vi "PV Calc.vi"(8 "error in (no error)":errorcluster, 11 "LimitControl in":refnum<class "LimitControl.lvclass">) -> (0 "error out":errorcluster, 3 "LimitControl out":refnum<class "LimitControl.lvclass">)   [LabVIEW 2020, in "VolatusControl.lvlib" / "LimitControl.lvclass"]
uses:
  LimitControl.lvclass
  LimitControl.lvclass/LimitControl.ctl
  lv-vecto/Vecto/Channel DBL/Channel DBL.lvclass/Channel DBL.ctl
  <vilib>/Analysis/baseanly.llb/Mean (DBL).vi
  lv-vecto/Vecto/Group DBL/Value by Index.vi
  lv-vecto/Vecto/Channel DBL/Channel DBL.lvclass
  <vilib>/Analysis/NI_AALBase.lvlib
panel:
  out "PV":dbl
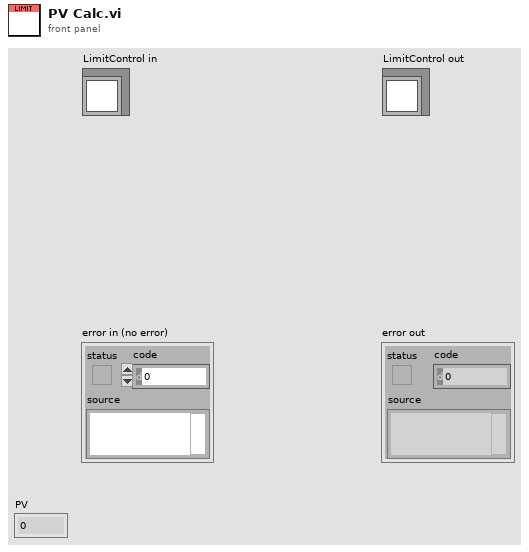
[diagram p1: front panel]
types:
  T1 = typedef "VolatusControl.lvlib/LimitControl.lvclass/PV Calc.ctl" = enum16{"Average", "Median"}
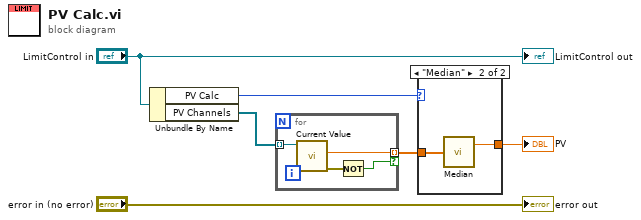
[diagram p0: block diagram]
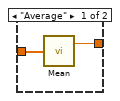
[diagram p2: hidden frame]
diagram:
  n1 = Unbundle By Name("LimitControl in") -> ("PV Calc"=w3:T1, "PV Channels"=w5:refnum<class "Channel DBL.lvclass">[])
  n2 = for {
    tunnel: w5 -> [w10] mode=indexing
    tunnel: [w9] -> w4 mode=indexing if=w7
    n3 = call "Current Value.vi"("Channel in"=w10) -> ("error out"=w8:errorcluster, "Scaled"=w9:dbl)  [unwired: 6 in, 3 out]
    n4 = Not(x=w8) -> (.not. x?=w7:bool)
  }
  n5 = case shown="\"Median\"" w3 {
    tunnel: w4 -> [w12 w14]
    tunnel: [w11 w13] -> w2
    frame "Average" {
      n6 = call-poly <vilib>:"Mean.vi"("X"=w12) -> ("mean"=w11:dbl)  [unwired: 1 out]
    }
    frame "Median" {
      n7 = call <vilib>:"Median.vi"("X"=w14) -> ("median"=w13:dbl)  [unwired: 1 out]
    }
  }
  "PV" <- w2
  "error out" <- "error in (no error)"
  "LimitControl out" <- "LimitControl in"
